vi "Get Rnd_User Input.vi"(8 "error in":errorcluster caption="에러 입력(에러 없음)") -> (0 "error out":errorcluster caption="에러 출력", 1 "변경?":bool, 2 "분해능 기준?":bool, 3 "0점 포함?":bool, 4 "조정후?":bool, 5 "1열 제외?":bool, 6 "조정전?":bool, 7 "변화량":dbl)   [LabVIEW 2020]
panel:
  in  "조정후":bool
  in  "조정전":bool
  in  "1열 제외":bool
  in  "0점 포함":bool
  in  "분해능 기준":bool=TRUE
  in  "입력값 기준":bool
  in  "확인":bool
  in  "변화량":dbl
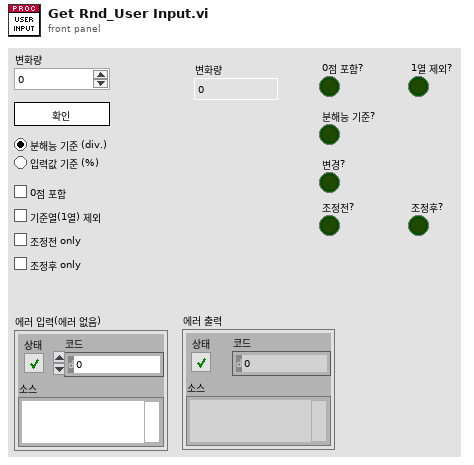
[diagram p1: front panel]
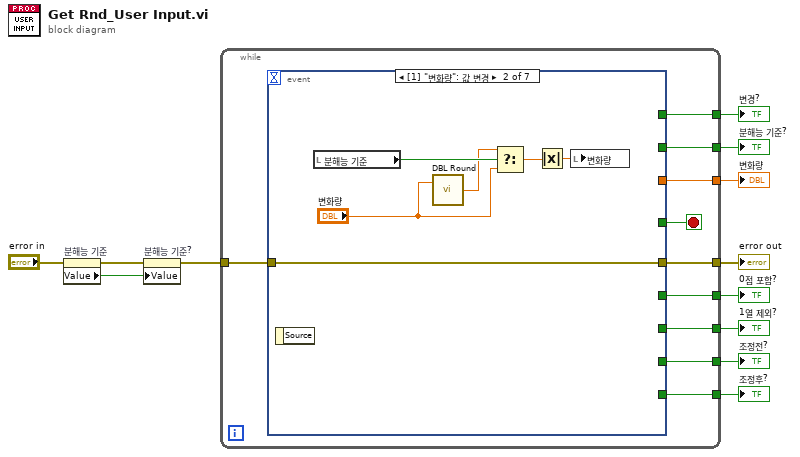
[diagram p0: block diagram]
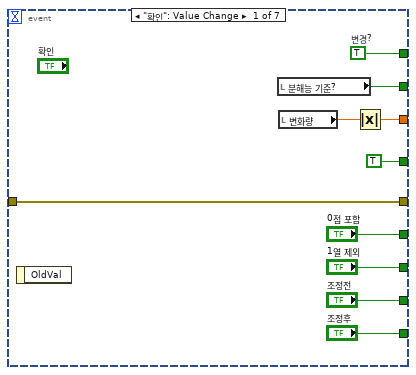
[diagram p2: hidden frame]
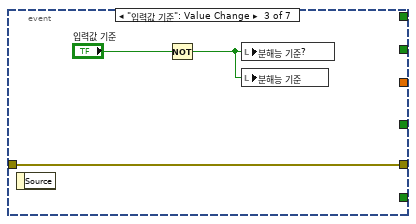
[diagram p3: hidden frame]
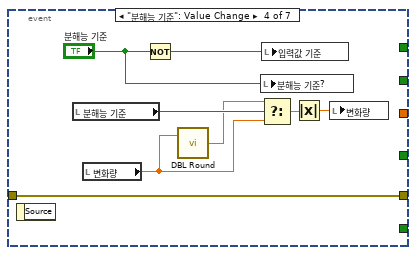
[diagram p4: hidden frame]
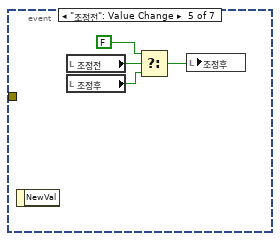
[diagram p5: hidden frame]
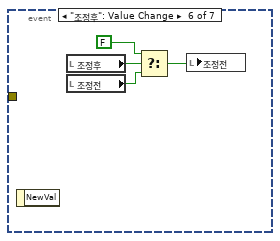
[diagram p6: hidden frame]
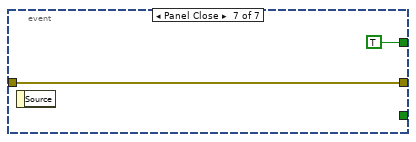
[diagram p7: hidden frame]
diagram:
  n1 = property on="분해능 기준" class="Bool (엄격한)"(error in="error in") -> (error out=w6:errorcluster, "Value"=w5:bool)  [unwired: 1 in, 1 out]
  n2 = property on="분해능 기준?" class="Bool (엄격한)"(error in=w6, "Value"=w5) -> (error out=w7:errorcluster)  [unwired: 1 in, 1 out]
  n3 = while {
    tunnel: [w19] -> w12
    tunnel: w7 -> [w20]
    tunnel: [w22] -> w11
    tunnel: [w18] -> w10
    tunnel: [w17] -> w9
    tunnel: [w16] -> w4
    tunnel: [w15] -> w3
    tunnel: [w14] -> w2
    tunnel: [w13] -> w1
    stop <- w21 stop-if-true
    n4 = event shown="[1] \"변화량\": 값 변경" {
      selector: _ -> [_ _ _ _ _ _ _]
      dyn-events: _ -> [_ _ _ _ _ _ _]
      timeout: _ -> [_ _ _ _ _ _ _]
      tunnel: [w25 _ _ _ _ _ _] -> w22
      tunnel: [TRUE ("확인") _ _ _ _ _ TRUE ("확인")] -> w21
      tunnel: w20 -> [w32 w38 w40 w49 _ _ w58]
      tunnel: [w32 w38 w40 w49 _ _ w58] -> w19
      tunnel: [w30 _ _ _ _ _ _] -> w18
      tunnel: [w29 _ _ _ _ _ _] -> w17
      tunnel: ["0점 포함" _ _ _ _ _ _] -> w16
      tunnel: ["1열 제외" _ _ _ _ _ _] -> w15
      tunnel: ["조정전" _ _ _ _ _ _] -> w14
      tunnel: ["조정후" _ _ _ _ _ _] -> w13
      event "확인": Value Change {
        w30 = TRUE  # 변경?
        n5 = event-data() -> ()  [unwired: 1 in, 1 out]
        n6 = local read "분해능 기준?"() -> (w29:bool)
        n7 = local read "변화량"() -> (w26:dbl)
        n8 = Absolute Value(x=w26) -> (abs(x)=w25:dbl)
      }
      event "변화량": Value Change {
        n9 = event-data() -> ()  [unwired: 1 in, 1 out]
        n10 = local read "분해능 기준"() -> (w37:bool)
        n11 = call "DBL Round.vi"("DBL in"="변화량") -> ("DBL out"=w33:dbl)  [unwired: 2 in]
        n12 = Select(t=w33, s=w37, f="변화량") -> (s? t:f=w36:dbl)
        n13 = Absolute Value(x=w36) -> (abs(x)=w35:dbl)
        n14 = local write "변화량"(w35) -> ()
      }
      event "입력값 기준": Value Change {
        n15 = event-data() -> ()  [unwired: 1 in, 1 out]
        n16 = Not(x="입력값 기준") -> (.not. x?=w39:bool)
        n17 = local write "분해능 기준?"(w39) -> ()
        n18 = local write "분해능 기준"(w39) -> ()
      }
      event "분해능 기준": Value Change {
        n19 = event-data() -> ()  [unwired: 1 in, 1 out]
        n20 = local read "분해능 기준"() -> (w46:bool)
        n21 = local read "변화량"() -> (w43:dbl)
        n22 = Not(x="분해능 기준") -> (.not. x?=w48:bool)
        n23 = call "DBL Round.vi"("DBL in"=w43) -> ("DBL out"=w42:dbl)  [unwired: 2 in]
        n24 = local write "분해능 기준?"("분해능 기준") -> ()
        n25 = local write "입력값 기준"(w48) -> ()
        n26 = Select(t=w42, s=w46, f=w43) -> (s? t:f=w45:dbl)
        n27 = Absolute Value(x=w45) -> (abs(x)=w44:dbl)
        n28 = local write "변화량"(w44) -> ()
      }
      event "조정전": Value Change {
        n29 = event-data() -> ()  [unwired: 1 in, 1 out]
        n30 = local read "조정전"() -> (w53:bool)
        n31 = local read "조정후"() -> (w50:bool)
        n32 = Select(t=FALSE ("조정후?"), s=w53, f=w50) -> (s? t:f=w51:bool)
        n33 = local write "조정후"(w51) -> ()
      }
      event "조정후": Value Change {
        n34 = event-data() -> ()  [unwired: 1 in, 1 out]
        n35 = local read "조정후"() -> (w57:bool)
        n36 = local read "조정전"() -> (w54:bool)
        n37 = Select(t=FALSE ("조정후?"), s=w57, f=w54) -> (s? t:f=w55:bool)
        n38 = local write "조정전"(w55) -> ()
      }
      event Panel Close {
        n39 = event-data() -> ()  [unwired: 1 in, 1 out]
      }
    }
  }
  "error out" <- w12
  "변화량" <- w11
  "변경?" <- w10
  "분해능 기준?" <- w9
  "0점 포함?" <- w4
  "1열 제외?" <- w3
  "조정전?" <- w2
  "조정후?" <- w1
